vi "datos usuario.vi"() -> ()   [LabVIEW 2018]
panel:
  in  "categoria":string
  in  "usuario":string
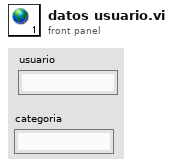
[diagram p1: front panel]
diagram:
